vi "vending_machine_events.vi"() -> ()   [LabVIEW 2018]
panel:
  out "next / stato":i32
  in  "B_Annulla":bool
  out "current time":timestamp
  out "messaggio":string
  out "somma":dbl
  out "resto":dbl
  in  "succo 0,60":bool
  in  "biscotti 1":bool
  in  "thè 0,35":bool
  in  "caffè 0,40":bool
  in  "#monete da 2":u8
  in  "#monete da 1":u8
  in  "#monete da 0,50":u8
  in  "#monete da 0,20":u8
  in  "#monete da 0,10":u8
  # "2"
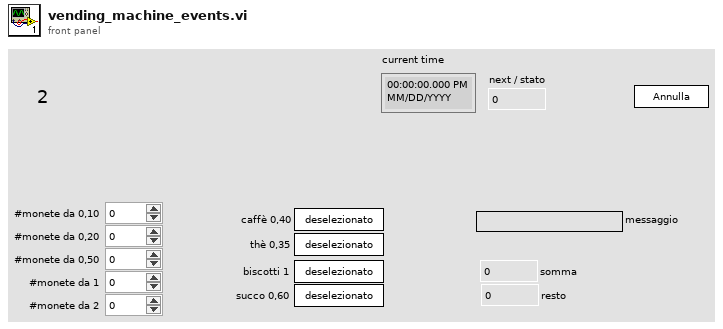
[diagram p1: front panel]
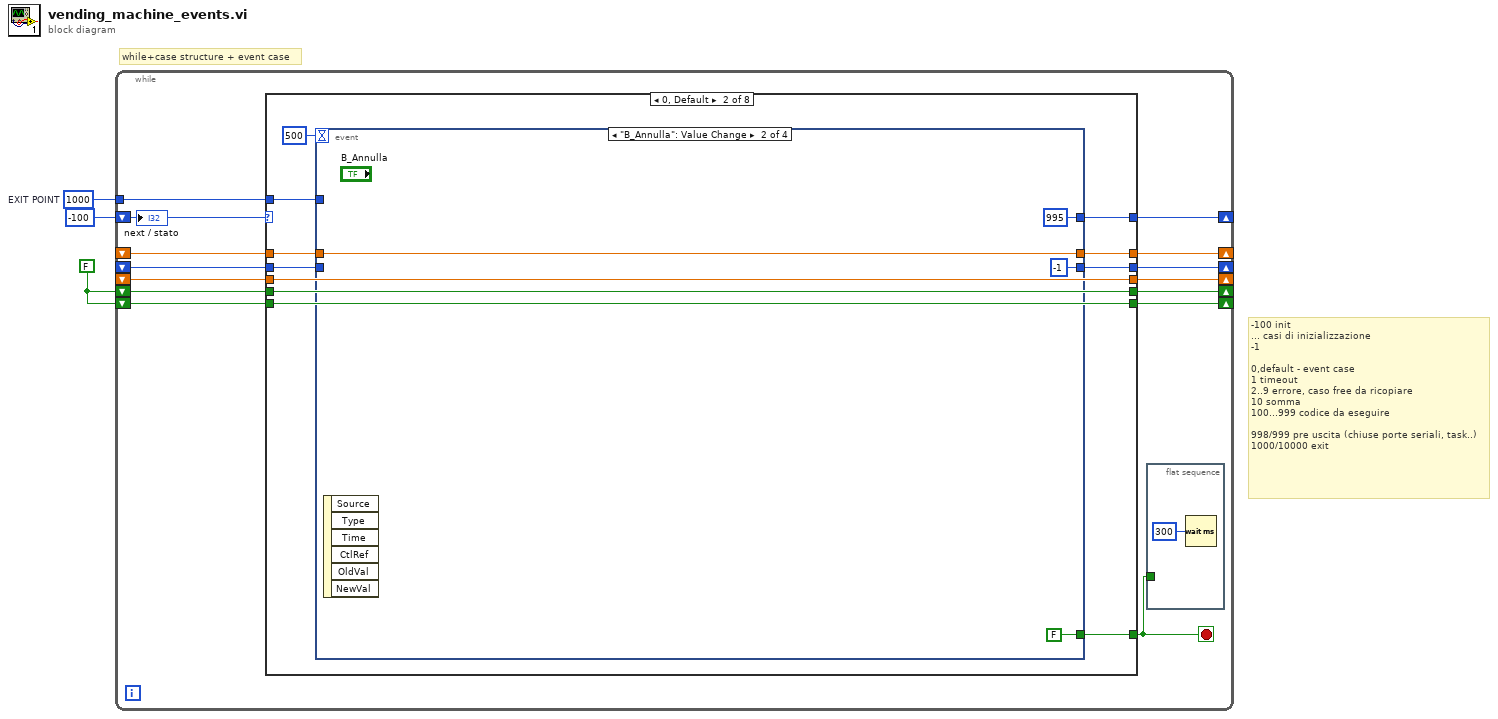
[diagram p0: block diagram]
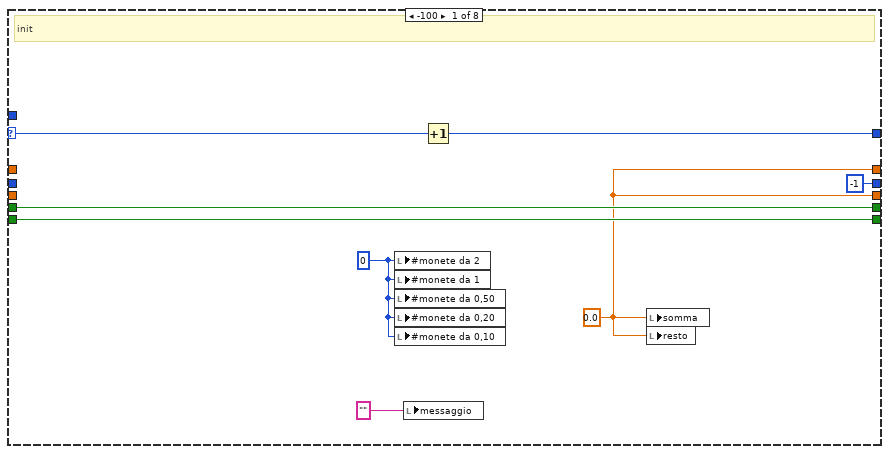
[diagram p2: hidden frame]
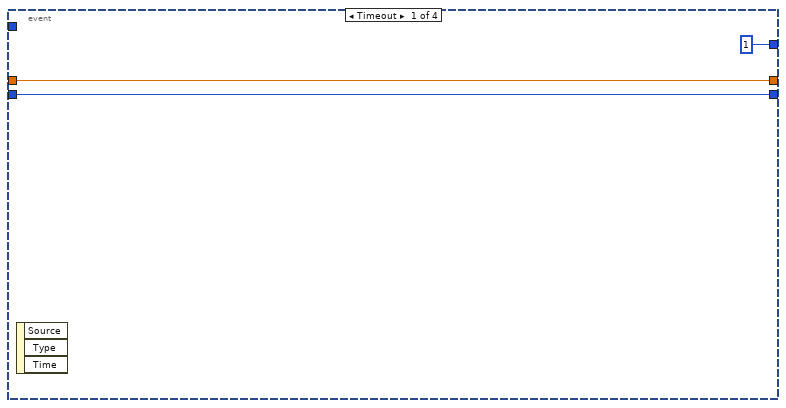
[diagram p3: hidden frame]
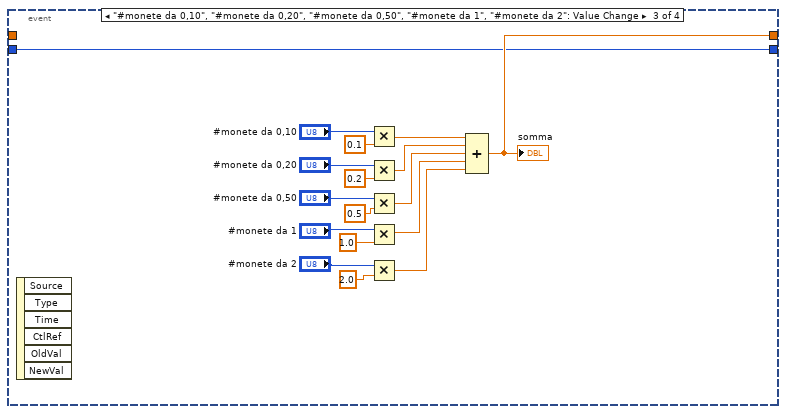
[diagram p4: hidden frame]
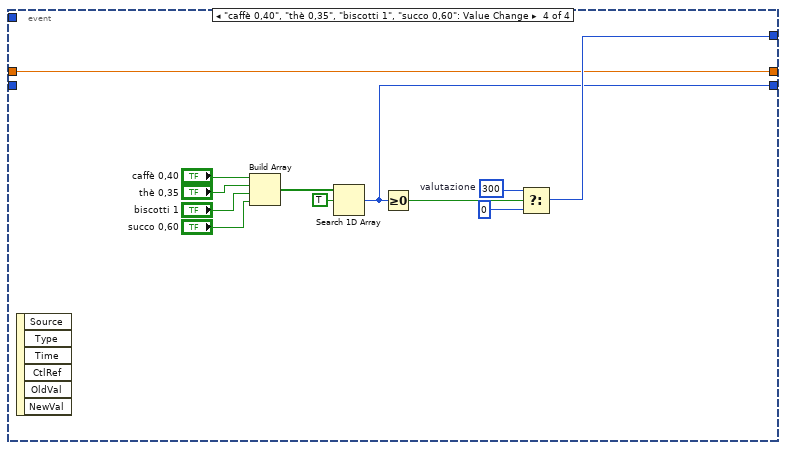
[diagram p5: hidden frame]
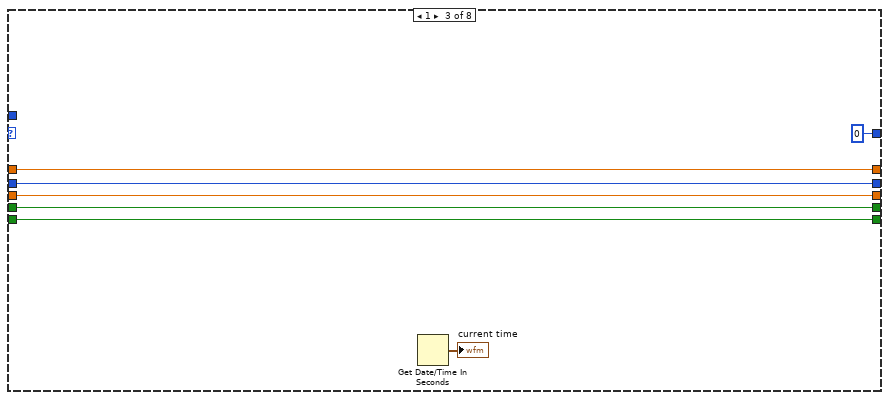
[diagram p6: hidden frame]
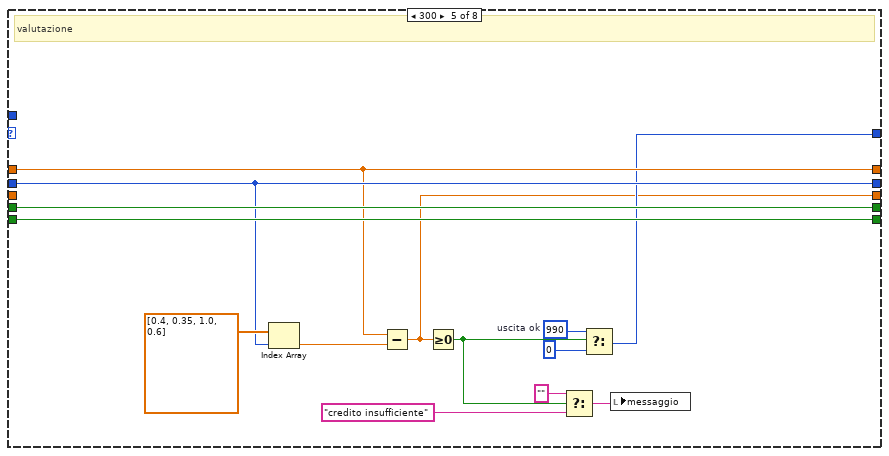
[diagram p8: hidden frame]
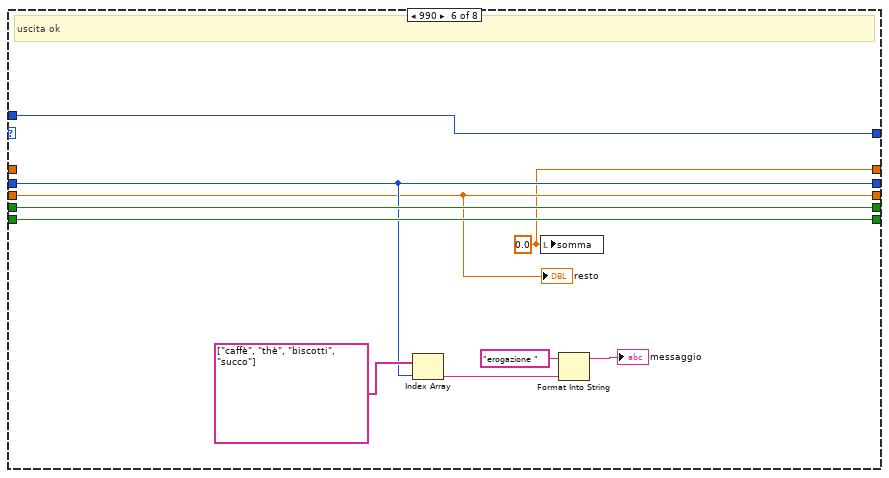
[diagram p9: hidden frame]
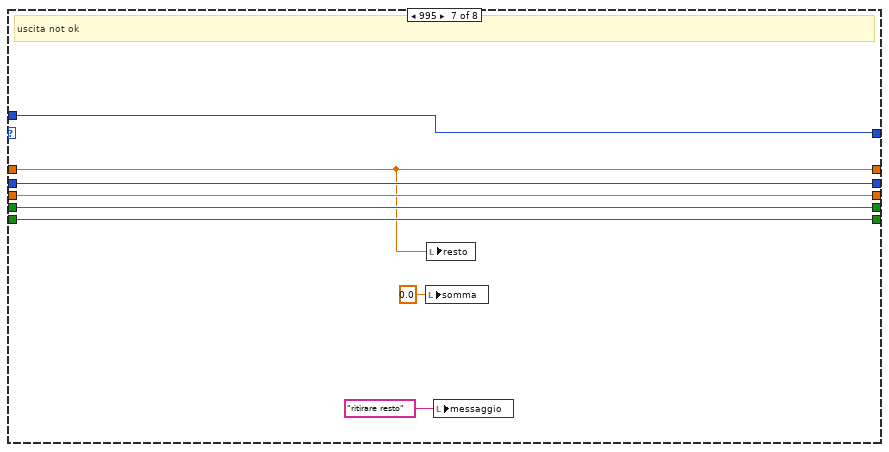
[diagram p10: hidden frame]
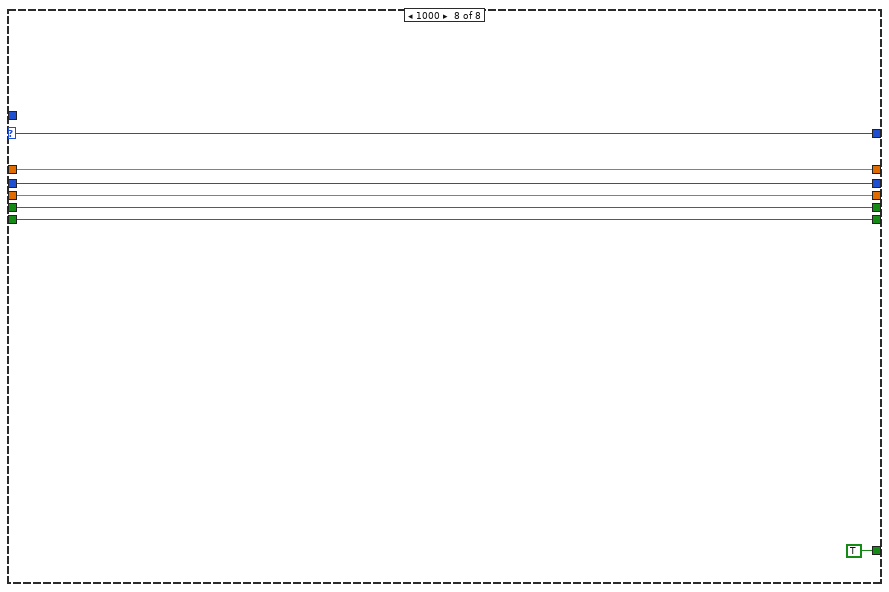
[diagram p11: hidden frame]
diagram:
  w1 = 1000  # EXIT POINT
  w2 = FALSE
  # "while+case structure + event case"
  # "-100 init\n... casi di inizializzazione\n-1\n\n0,default - event case\n1 timeout\n2..9 errore, caso free da ricopiare\n10 somma\n100...999 codice da eseguire\n\n998/999 pre uscita (chiuse porte seriali, task..)\n1000/10000 exit"
  n1 = while {
    shift-right: [w17] -> _
    shift-left: -100 -> [w6]
    shift-right: [w15] -> _
    shift-left: _ -> [w16]
    shift-right: [w13] -> _
    shift-left: _ -> [w14]
    shift-right: [w11] -> _
    shift-left: _ -> [w12]
    shift-right: [w9] -> _
    shift-left: w2 -> [w10]
    shift-right: [w7] -> _
    shift-left: w2 -> [w8]
    tunnel: w1 -> [w5]
    stop <- w4 stop-if-true
    n2 = case shown="0, Default" w6 {
      selector: w6 -> [w23 _ _ w86 _ _ _ w119]
      tunnel: [w26 w36 0 w86 w90 w102 w114 w119] -> w17
      tunnel: w16 -> [_ w28 w78 w85 w91 _ w112 w125]
      tunnel: [w20 w30 w78 w85 w91 w101 w112 w125] -> w15
      tunnel: [-1 ("index of element") w29 w77 w84 w92 w104 w118 w124] -> w13
      tunnel: w14 -> [_ w27 w77 w84 w92 w104 w118 w124]
      tunnel: w12 -> [_ w35 w76 w83 _ w103 w117 w123]
      tunnel: [w20 w35 w76 w83 w87 w103 w117 w123] -> w11
      tunnel: w10 -> [w25 w34 w75 w82 w100 w110 w116 w122]
      tunnel: [w25 w34 w75 w82 w100 w110 w116 w122] -> w9
      tunnel: w8 -> [w24 w33 w74 w81 w99 w109 w115 w121]
      tunnel: [w24 w33 w74 w81 w99 w109 w115 w121] -> w7
      tunnel: [_ w32 _ _ _ _ _ TRUE] -> w4
      tunnel: w5 -> [_ w31 _ _ _ w102 w114 _]
      frame -100 {
        w20 = 0.0 ("somma")
        w21 = u8 0 ("#monete da 2")
        # "init"
        n3 = local write "#monete da 2"(w21) -> ()
        n4 = local write "#monete da 1"(w21) -> ()
        n5 = local write "#monete da 0,50"(w21) -> ()
        n6 = local write "#monete da 0,20"(w21) -> ()
        n7 = local write "#monete da 0,10"(w21) -> ()
        n8 = local write "messaggio"("" ("articolo scelto")) -> ()
        n9 = Increment(x=w23) -> (x+1=w26:i32)
        n10 = local write "somma"(w20) -> ()
        n11 = local write "resto"(w20) -> ()
      }
      frame 0, Default {
        n12 = event shown="[1] \"B_Annulla\": Value Change" {
          selector: _ -> [_ _ _ _]
          dyn-events: _ -> [_ _ _ _]
          timeout: 500 -> [_ _ _ _]
          tunnel: [1 995 ("valutazione") _ w64] -> w36
          tunnel: [_ FALSE _ _] -> w32
          tunnel: w31 -> [_ _ _ _]
          tunnel: [w39 w43 w46 w62] -> w30
          tunnel: [w38 -1 ("index of element") w45 w63] -> w29
          tunnel: w28 -> [w39 w43 _ w62]
          tunnel: w27 -> [w38 _ w45 _]
          event Timeout {
            n13 = event-data() -> ()  [unwired: 1 in, 3 out]
          }
          event "B_Annulla": Value Change {
            n14 = event-data() -> ()  [unwired: 1 in, 6 out]
          }
          event "#monete da 0,10", "#monete da 0,20", "#monete da 0,50", "#monete da 1", "#monete da 2": Value Change {
            n15 = event-data() -> ()  [unwired: 1 in, 6 out]
            n16 = Multiply(x="#monete da 0,10", y=0.1) -> (x*y=w52:dbl)
            n17 = Multiply(x="#monete da 0,20", y=0.2) -> (x*y=w58:dbl)
            n18 = Multiply(x="#monete da 0,50", y=0.5) -> (x*y=w59:dbl)
            n19 = Multiply(x="#monete da 1", y=1.0) -> (x*y=w60:dbl)
            n20 = Multiply(x="#monete da 2", y=2.0) -> (x*y=w61:dbl)
            n21 = Compound Arithmetic op=ADD(w52, w58, w59, w60, w61) -> (w46:dbl)
            "somma" <- w46
          }
          event "caffè 0,40", "thè 0,35", "biscotti 1", "succo 0,60": Value Change {
            w66 = 300  # valutazione
            n22 = event-data() -> ()  [unwired: 1 in, 6 out]
            n23 = Build Array("caffè 0,40", "thè 0,35", "biscotti 1", "succo 0,60") -> (w72:bool[])
            n24 = Search 1D Array(1D array=w72, element=TRUE) -> (index of element=w63:i32)  [unwired: 1 in]
            n25 = Greater Or Equal To 0?(x=w63) -> (x >= 0?=w73:bool)
            n26 = Select(t=w66, s=w73, f=0) -> (s? t:f=w64:i32)
          }
        }
      }
      frame 1 {
        n27 = Get Date/Time In Seconds() -> (seconds since 1Jan1904=→"current time":timestamp)
      }
      frame 3 {
        # "free"
      }
      frame 300 {
        w89 = 990  # uscita ok
        # "valutazione"
        n28 = Index Array(array=dbl[] [0.4, 0.35, 1.0, 0.6], index=w92) -> (element=w94:dbl)
        n29 = Subtract(x=w91, y=w94) -> (x-y=w87:dbl)
        n30 = Greater Or Equal To 0?(x=w87) -> (x >= 0?=w95:bool)
        n31 = Select(t="", s=w95, f="credito insufficiente" ("messaggio")) -> (s? t:f=w96:string)
        n32 = Select(t=w89, s=w95, f=0) -> (s? t:f=w90:i32)
        n33 = local write "messaggio"(w96) -> ()
      }
      frame 990 {
        w101 = 0.0 ("somma")
        # "uscita ok"
        n34 = Index Array(array=string[] ["caffè", "thè", "biscotti", "succo"], index=w104) -> (element=w107:string)
        n35 = local write "somma"(w101) -> ()
        n36 = Format Into String(initial string="erogazione ", w107) -> (resulting string=→"messaggio":string)  [unwired: 2 in, 1 out]
        "resto" <- w103
      }
      frame 995 {
        # "uscita not ok"
        n37 = local write "somma"(0.0 ("somma")) -> ()
        n38 = local write "resto"(w112) -> ()
        n39 = local write "messaggio"("ritirare resto" ("articolo scelto")) -> ()
      }
      frame 1000 {
      }
    }
    n40 = flat-sequence {
      tunnel: w4 -> [_]
      frame #0 {
        n41 = Wait (ms)(milliseconds to wait=u32 300) -> ()  [unwired: 1 out]
      }
    }
    "next / stato" <- w6
  }
